vi "bias_on_off_int.vi"() -> ()   [LabVIEW 2011]
panel:
  in  "Frequency":dbl
  out "STATE":bool
  in  "STOP":bool
  out "error out":errorcluster
  out "VISA Out":refnum<visa-resource-name>
  in  "VISA In":refnum<visa-resource-name>
  in  "error in (no error)":errorcluster
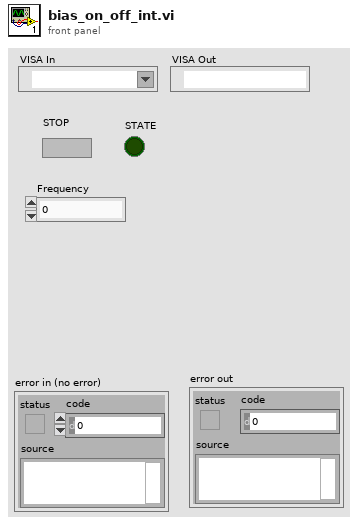
[diagram p1: front panel]
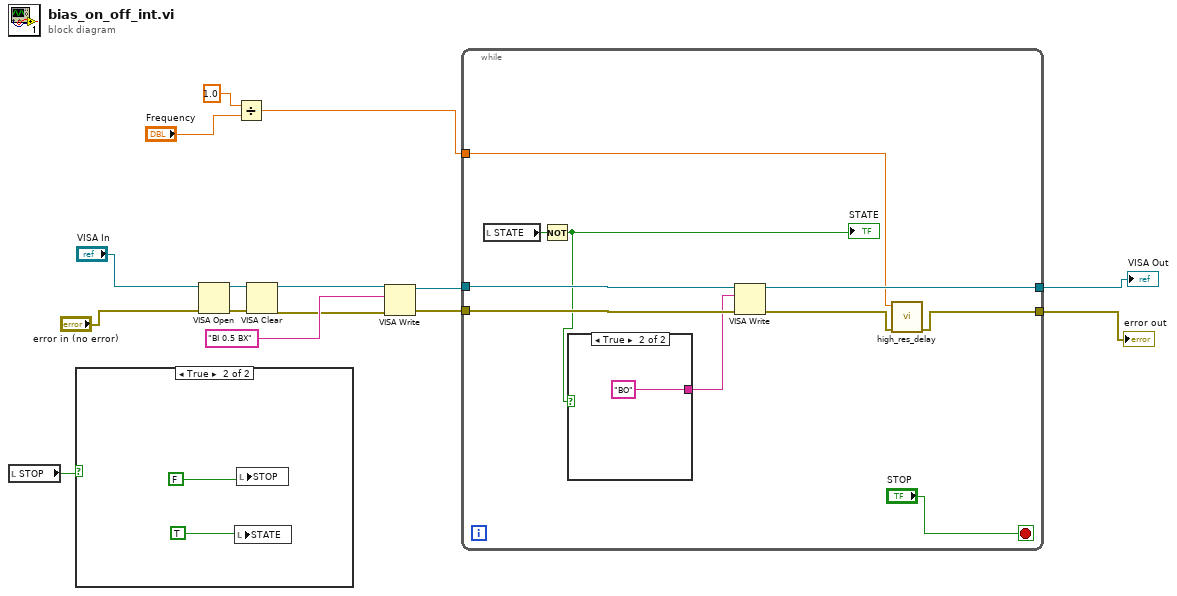
[diagram p0: block diagram]
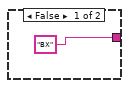
[diagram p3: hidden frame]
diagram:
  n1 = local read "STOP"() -> (w13:bool)
  n2 = case shown="True" w13 {
    frame False {
    }
    frame True {
      n3 = local write "STATE"(TRUE) -> ()
      n4 = local write "STOP"(FALSE) -> ()
    }
  }
  n5 = VISA Open(error in (no error)="error in (no error)", VISA resource name="VISA In") -> (VISA resource name=w14:refnum<visa-resource-name>, error out=w15:errorcluster)  [unwired: 3 in]
  n6 = Divide(x=1.0, y="Frequency") -> (x/y=w6:dbl)
  n7 = VISA Clear(VISA resource name=w14, error in (no error)=w15) -> (VISA resource name out=w2:refnum<visa-resource-name>, error out=w1:errorcluster)
  n8 = VISA Write(VISA resource name=w2, write buffer="BI 0.5 BX", error in (no error)=w1) -> (VISA resource name out=w5:refnum<visa-resource-name>, error out=w4:errorcluster)  [unwired: 1 out]
  n9 = while {
    tunnel: w5 -> [w27]
    tunnel: w4 -> [w26]
    tunnel: [w22] -> w10
    tunnel: [w21] -> w9
    tunnel: w6 -> [w19]
    stop <- "STOP" stop-if-true
    n10 = local read "STATE"() -> (w24:bool)
    n11 = Not(x=w24) -> (.not. x?=w18:bool)
    "STATE" <- w18
    n12 = case shown="True" w18 {
      tunnel: ["BX" "BO"] -> w23
      frame False {
      }
      frame True {
      }
    }
    n13 = VISA Write(VISA resource name=w27, write buffer=w23, error in (no error)=w26) -> (VISA resource name out=w22:refnum<visa-resource-name>, error out=w20:errorcluster)  [unwired: 1 out]
    n14 = call "high_res_delay.vi"("error in (no error)"=w20, "Delay (sec)"=w19) -> ("error out"=w21:errorcluster)  [unwired: 9 in]
  }
  "VISA Out" <- w10
  "error out" <- w9
